vi "Get Database Item Types.vi"(8 "error in (no error)":errorcluster, 11 "eLab in":refnum<class "PL eLabFTW Client.lvclass">) -> (0 "error out":errorcluster, 2 "types":T1(array[cluster]), 3 "eLab out":refnum<class "PL eLabFTW Client.lvclass">)   [LabVIEW 2015, in "PL eLabFTW Client.lvclass"]
doc: "Gets database item types."
uses:
  PL eLabFTW Client.lvclass
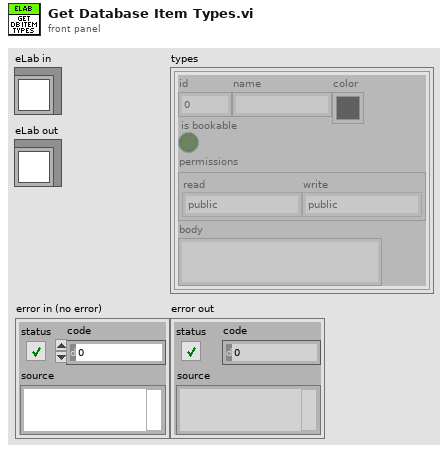
[diagram p1: front panel]
types:
  T1 = cluster{"id":u32, "name":string, "color":u32, "is bookable":bool, "permissions":cluster{"read":enum16{"public", "organization", "team", "owner and admins", "owner"}, "write":enum16{"public", "organization", "team", "owner and admins", "owner"}}, "body":string}[]
  T2 = cluster{"category_id":string, "category":string, "color":string, "bookable":string, "body":string, "ordering":string, "canread":string, "canwrite":string}[]
  T3 = cluster{"id":u32, "name":string, "color":u32, "is bookable":bool, "permissions":cluster{"read":enum16{"public", "organization", "team", "owner and admins", "owner"}, "write":enum16{"public", "organization", "team", "owner and admins", "owner"}}, "body":string}
  T4 = enum16{"public", "organization", "team", "owner and admins", "owner"}
  T5 = cluster{"category_id":i32, "category":i32, "color":i32, "bookable":i32, "body":i32, "ordering":i32, "canread":i32, "canwrite":i32}
  T6 = cluster{"category_id":bool, "category":bool, "color":bool, "bookable":bool, "body":bool, "ordering":bool, "canread":bool, "canwrite":bool}
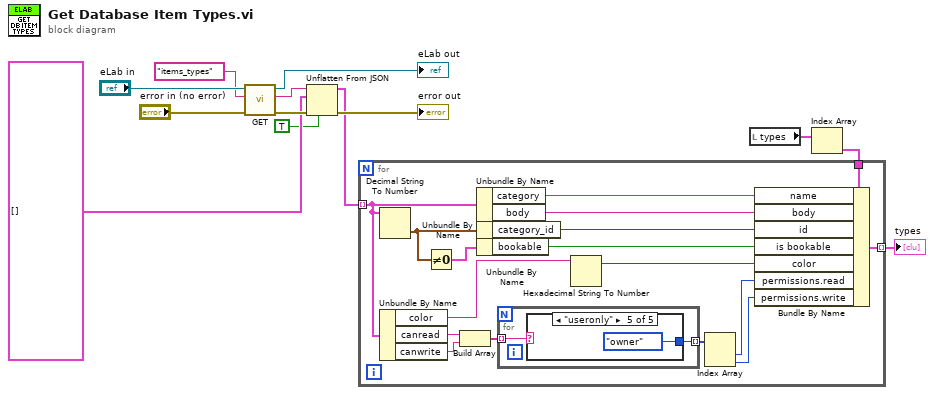
[diagram p0: block diagram]
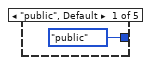
[diagram p2: hidden frame]
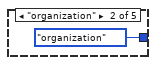
[diagram p3: hidden frame]
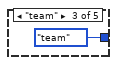
[diagram p4: hidden frame]
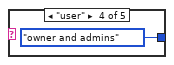
[diagram p5: hidden frame]
diagram:
  n1 = call "GET.vi"("error in (no error)"="error in (no error)", "relative URL"="items_types", "eLab in"="eLab in") -> ("error out"=w8:errorcluster, "response body"=w9:string, "eLab out"=→"eLab out":refnum<class "PL eLabFTW Client.lvclass">)  [unwired: 6 in]
  n2 = Unflatten From JSON(JSON string=w9, type and defaults=T2 [], default null elements? (F)=TRUE, error in (no error)=w8) -> (value=w5:T2, error out=→"error out":errorcluster)  [unwired: 3 in]
  n3 = local read "types"() -> (w4:T1)
  n4 = Index Array(array=w4) -> (element=w3:T3)  [unwired: 1 in]
  n5 = for {
    tunnel: w5 -> [w23] mode=indexing
    tunnel: w3 -> [w16]
    tunnel: [w30] -> w2 mode=indexing
    n6 = Decimal String To Number(string=w23) -> (number=w27:T5)  [unwired: 2 in, 1 out]
    n7 = Unbundle By Name(w23) -> ("color"=w18:string, "canread"=w22:string, "canwrite"=w21:string)
    n8 = Not Equal To 0?(x=w27) -> (x != 0?=w26:T6)
    n9 = Build Array(w22, w21) -> (w20:string[])
    n10 = Unbundle By Name(w23) -> ("category"=w29:string, "body"=w28:string)
    n11 = Unbundle By Name(w27) -> ("category_id"=w25:i32)
    n12 = Unbundle By Name(w26) -> ("bookable"=w24:bool)
    n13 = for {
      tunnel: w20 -> [w32] mode=indexing
      tunnel: [w31] -> w19 mode=indexing
      n14 = case shown="\"useronly\"" w32 {
        tunnel: [T4."public" ("permissions.read") T4."organization" ("permissions.read") T4."team" ("permissions.read") T4."owner and admins" ("permissions.read") T4."owner" ("permissions.read")] -> w31
        frame "public", Default {
        }
        frame "organization" {
        }
        frame "team" {
        }
        frame "user" {
        }
        frame "useronly" {
        }
      }
    }
    n15 = Hexadecimal String To Number(string=w18) -> (offset past number=w17:i32)  [unwired: 2 in, 1 out]
    n16 = Index Array(array=w19) -> (element #1=w15:T4, element #2=w14:T4)  [unwired: 2 in]
    n17 = Bundle By Name(cluster=w16, "name"=w29, "body"=w28, "id"=w25, "is bookable"=w24, "color"=w17, "permissions.read"=w15, "permissions.write"=w14) -> (w30:T3)
  }
  "types" <- w2
